vi "P4CMD Is File In Local Path.vi"(8 "error in (no error)":errorcluster, 10 "files":path[](array[path]), 11 "source control reference in":T1) -> (0 "error out":errorcluster, 2 "in local path?":bool[](array[boolean]), 3 "source control reference out":T1)   [LabVIEW 2020, in "NI_SCC_P4CMD.lvlib"]
uses:
  <vilib>/SourceControl/Providers/P4CMD/NI_SCC_P4CMD.lvlib
  <vilib>/SourceControl/sccapi/SCCAPI Refnum.ctl
  <vilib>/SourceControl/Providers/P4CMD/P4CMD Operations.ctl
  <vilib>/SourceControl/sccapi/NI_SCC.lvlib
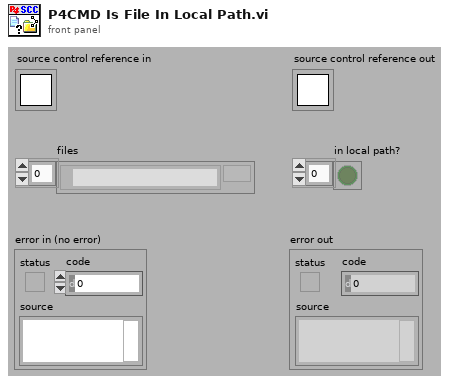
[diagram p1: front panel]
types:
  T1 = typedef "NI_SCC.lvlib/SCCAPI Refnum.ctl" = refnum<k1>
  T2 = typedef "NI_SCC_P4CMD.lvlib/P4CMD Operations.ctl" = enum16{"get all clients", "get all users", "describe changelist", "sync from depot", "open for edit", "submit to depot", "revert", "add to depot", "remove from depot", "print files revisions", "compare client file", "print depot file contents", "list opened files", "get file info", "lock files", "edit changelist spec", "info", "set variables"}
  T3 = enum32{"invalid OS target", "Mac OS", "Windows 3.1", "Windows 95/NT", "Solaris 1", "Solaris 2", "HP-UX", "PowerMAX", "Linux", "Irix", "Rhapsody", "BeOS", "AIX", "OSF1", "VxWorks", "PharLap", "Carbon", "RTX", "Windows x64", "Linux x64", "Mac OS X x64"}
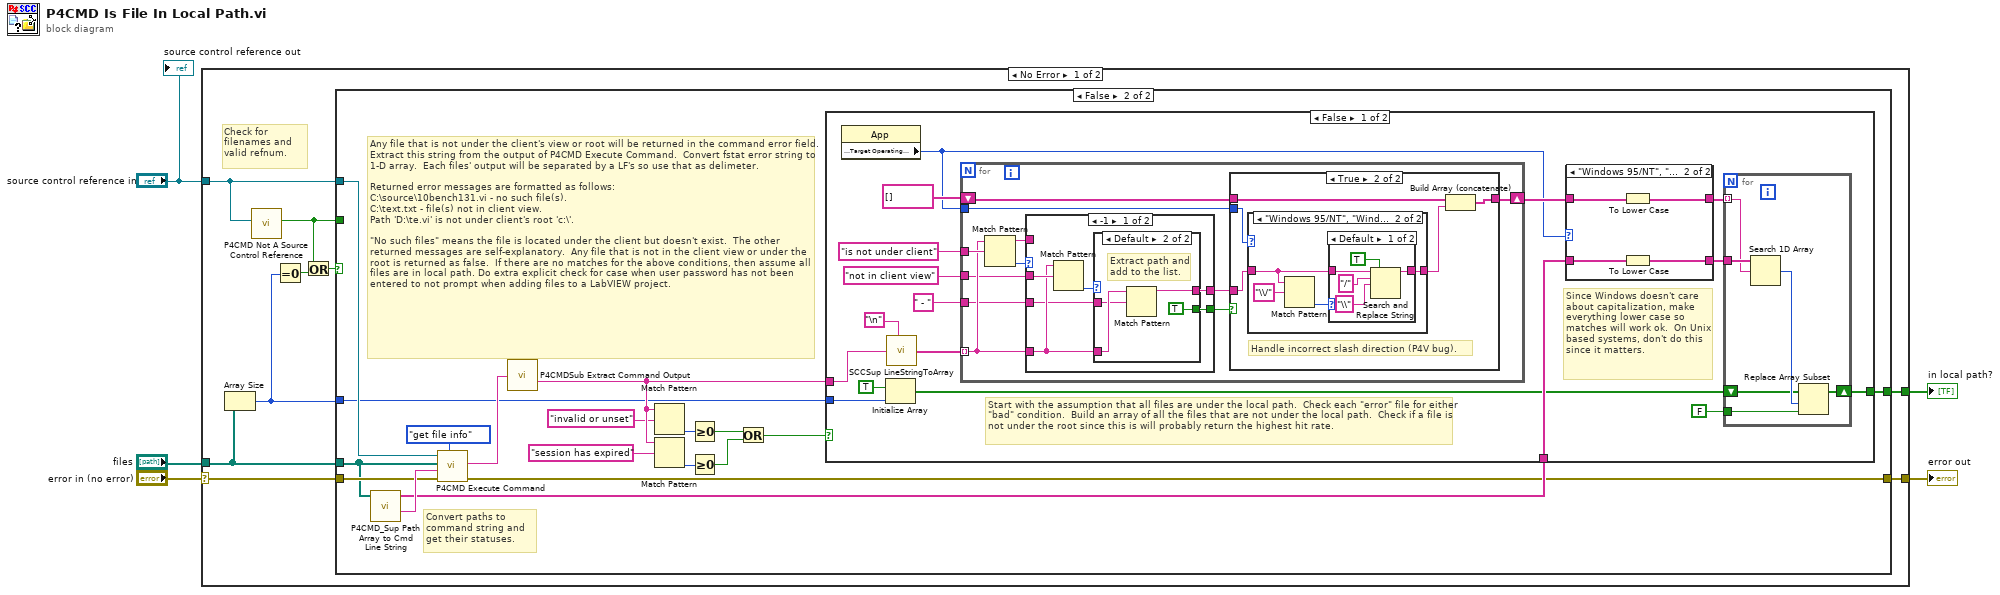
[diagram p0: block diagram]
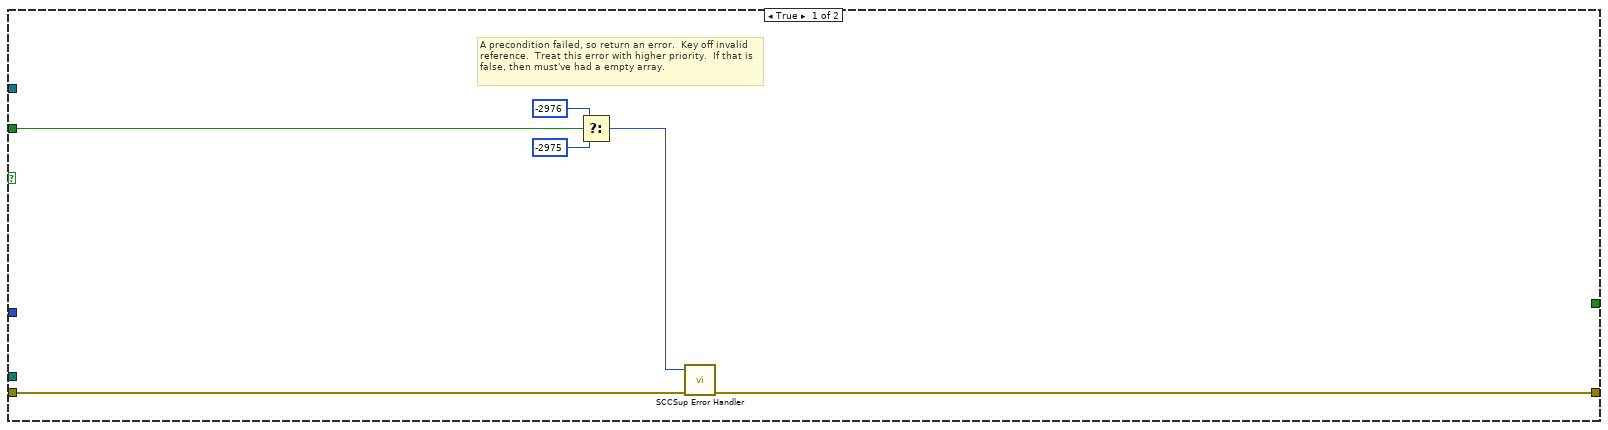
[diagram p2: hidden frame]
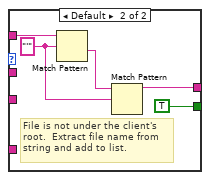
[diagram p5: hidden frame]
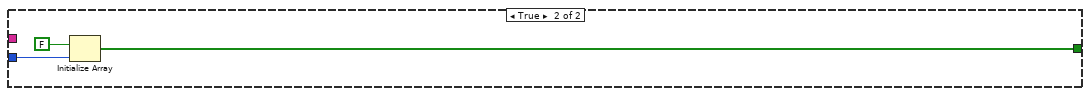
[diagram p9: hidden frame]
diagram:
  n1 = case shown="No Error" "error in (no error)" {
    selector: "error in (no error)" -> [w14 w114]
    tunnel: [w9 w114] -> w4
    tunnel: "files" -> [w11 _]
    tunnel: "source control reference in" -> [w12 _]
    tunnel: [w7 _] -> w1
    frame No Error {
      # "Check for filenames and valid refnum."
      n2 = Array Size(array=w11) -> (size(s)=w8:i32)
      n3 = call <vilib>:"P4CMD Not A Source Control Reference.vi"("source control reference in"=w12) -> ("not a source control reference?"=w6:bool)  [unwired: 9 in, 1 out]
      n4 = Equal To 0?(x=w8) -> (x = 0?=w13:bool)
      n5 = Or(x=w6, y=w13) -> (x .or. y?=w10:bool)
      n6 = case shown="False" w10 {
        tunnel: w14 -> [w17 w36]
        tunnel: w11 -> [_ w35]
        tunnel: w12 -> [_ w34]
        tunnel: w6 -> [w16 _]
        tunnel: [w15 w31] -> w9
        tunnel: w8 -> [_ w21]
        tunnel: [_ w30] -> w7
        frame True {
          # "A precondition failed, so return an error.  Key off invalid reference.  Treat this error with higher priority.  If that is false, then must've had a empty array."
          n7 = Select(t=-2976 ("result"), s=w16, f=-2975 ("result")) -> (s? t:f=w18:i32)
          n8 = call <vilib>:"SCCSup Error Handler.vi"("error in (no error)"=w17, "scc error code"=w18) -> ("error out"=w15:errorcluster)  [unwired: 9 in]
        }
        frame False {
          # "Convert paths to command string and get their statuses."
          # "Any file that is not under the client's view or root will be returned in the command error field.  Extract this string from the output of P4CMD Execute Command.  Convert fstat error string to 1-D array.  Each files' output will be separated by a LF's so use that as delimeter.\n\nReturned error messages are formatted as follows:\nC:\\source\\10bench131.vi - no such file(s).\nC:\\text.txt - file(s) not in client view.\nPath 'D:\\te.vi' is not under client's root 'c:\\'. \n\n\"No such files\" means the file is located under the client but doesn't exist.  The other returned messages are self-explanatory.  Any file that is not in the client view or under the root is returned as false.  If there are no matches for the above conditions, then assume all files are in local path. Do extra explicit check for case when user password has not been entered to not prompt when adding files to a LabVIEW project."
          n9 = call <vilib>:"P4CMD_Sup Path Array to Cmd Line String.vi"("files"=w35) -> ("string output"=w37:string, "converted file strings"=w32:string[])  [unwired: 9 in]
          n10 = call <vilib>:"P4CMD Execute Command.vi"("p4 operation"=P4CMD_Operations."get file info", "error in (no error)"=w36, "input string"=w37, "files"=w35, "source control reference in"=w34) -> ("error out"=w31:errorcluster, "command information"=w33:string)  [unwired: 4 in, 1 out]
          n11 = call <vilib>:"P4CMDSub Extract Command Output.vi"("bundled message"=w33) -> ("command error"=w25:string)  [unwired: 13 in, 1 out]
          n12 = Match Pattern(string=w25, regular expression="invalid or unset") -> (offset past match=w23:i32)  [unwired: 1 in, 3 out]
          n13 = Match Pattern(string=w25, regular expression="session has expired") -> (offset past match=w27:i32)  [unwired: 1 in, 3 out]
          n14 = Greater Or Equal To 0?(x=w23) -> (x >= 0?=w22:bool)
          n15 = Greater Or Equal To 0?(x=w27) -> (x >= 0?=w26:bool)
          n16 = Or(x=w22, y=w26) -> (x .or. y?=w28:bool)
          n17 = case shown="False" w28 {
            tunnel: w25 -> [w54 _]
            tunnel: w32 -> [w49 _]
            tunnel: [w46 w111] -> w30
            tunnel: w21 -> [w41 w112]
            frame False {
              # "Start with the assumption that all files are under the local path.  Check each \"error\" file for either \"bad\" condition.  Build an array of all the files that are not under the local path.  Check if a file is not under the root since this is will probably return the highest hit rate."
              # "Since Windows doesn't care about capitalization, make everything lower case so matches will work ok.  On Unix based systems, don't do this since it matters."
              n18 = property class="App"() -> ("Application:Target Operating System"=w39:T3)  [unwired: 2 in, 2 out]
              n19 = Initialize Array(TRUE, w41) -> (w40:bool[])
              n20 = call <vilib>:"SCCSup LineStringToArray.vi"("delimiter (Tab)"="\n", "line string"=w54) -> ("line array"=w53:string[])  [unwired: 7 in]
              n21 = for {
                tunnel: w53 -> [w71] mode=indexing
                tunnel: "is not under client" ("regular expression") -> [w78]
                shift-right: [w77] -> w50
                shift-left: string[] [] -> [w76]
                tunnel: "not in client view" ("regular expression") -> [w70]
                tunnel: " - " ("regular expression") -> [w69]
                tunnel: w39 -> [w68]
                n22 = Match Pattern(string=w71, regular expression=w78) -> (before substring=w74:string, offset past match=w75:i32)  [unwired: 1 in, 2 out]
                n23 = case shown="-1" w75 {
                  tunnel: w74 -> [_ w93]
                  tunnel: [w80 w90] -> w72
                  tunnel: [w79 TRUE] -> w73
                  tunnel: w71 -> [w82 _]
                  tunnel: w70 -> [w84 _]
                  tunnel: w69 -> [w81 _]
                  frame -1 {
                    n24 = Match Pattern(string=w82, regular expression=w84) -> (offset past match=w83:i32)  [unwired: 1 in, 3 out]
                    n25 = case shown="Default" w83 {
                      tunnel: w82 -> [_ w88]
                      tunnel: w81 -> [_ w87]
                      tunnel: [_ w86] -> w80
                      tunnel: [_ TRUE] -> w79
                      frame -1 {
                        # "There was an \"error\" but it was because the file was not found in the client view which is ok for this check."
                      }
                      frame Default {
                        # "Extract path and add to the list."
                        n26 = Match Pattern(string=w88, regular expression=w87) -> (before substring=w86:string)  [unwired: 1 in, 3 out]
                      }
                    }
                  }
                  frame Default {
                    w91 = "'" ("regular expression")
                    # "File is not under the client's root.  Extract file name from string and add to list."
                    n27 = Match Pattern(string=w93, regular expression=w91) -> (after substring=w92:string)  [unwired: 1 in, 3 out]
                    n28 = Match Pattern(string=w92, regular expression=w91) -> (before substring=w90:string)  [unwired: 1 in, 3 out]
                  }
                }
                n29 = case shown="True" w73 {
                  tunnel: w72 -> [_ w96]
                  tunnel: [w94 w99] -> w77
                  tunnel: w76 -> [w94 w98]
                  tunnel: w68 -> [_ w95]
                  frame False {
                  }
                  frame True {
                    # "Handle incorrect slash direction (P4V bug)."
                    n30 = case shown="\"Windows 95/NT\", \"Windows x64\"" w95 {
                      tunnel: [w100 w102] -> w97
                      tunnel: w96 -> [w100 w101]
                      frame "invalid OS target", Default {
                      }
                      frame "Windows 95/NT", "Windows x64" {
                        n31 = Match Pattern(string=w101, regular expression="\\/") -> (offset past match=w103:i32)  [unwired: 1 in, 3 out]
                        n32 = case shown="Default" w103 {
                          tunnel: w101 -> [w109 w110]
                          tunnel: [w105 w110] -> w102
                          frame Default {
                            n33 = Search and Replace String(replace all?=TRUE ("replace all? (F)"), input string=w109, search string="/" ("regular expression"), replace string="\\" ("regular expression")) -> (result string=w105:string)  [unwired: 4 in, 3 out]
                          }
                          frame -1 {
                          }
                        }
                      }
                    }
                    n34 = Build Array (concatenate)(w98, w97) -> (w99:string[])
                  }
                }
              }
              n35 = case shown="\"Windows 95/NT\", \"Windows x64\"" w39 {
                tunnel: w50 -> [w63 w67]
                tunnel: w49 -> [w62 w66]
                tunnel: [w63 w65] -> w47
                tunnel: [w62 w64] -> w48
                frame Default {
                }
                frame "Windows 95/NT", "Windows x64" {
                  n36 = To Lower Case(string=w67) -> (all lower case string=w65:string[])
                  n37 = To Lower Case(string=w66) -> (all lower case string=w64:string[])
                }
              }
              n38 = for {
                tunnel: w48 -> [w61]
                tunnel: w47 -> [w60] mode=indexing
                shift-right: [w57] -> w46
                shift-left: w40 -> [w58]
                tunnel: FALSE -> [w56]
                n39 = Search 1D Array(1D array=w61, element=w60) -> (index of element=w59:i32)  [unwired: 1 in]
                n40 = Replace Array Subset(array=w58, new element=w56, index=w59) -> (w57:bool[])
              }
            }
            frame True {
              n41 = Initialize Array(FALSE, w112) -> (w111:bool[])
            }
          }
        }
      }
    }
    frame Error {
    }
  }
  "error out" <- w4
  "in local path?" <- w1
  "source control reference out" <- "source control reference in"
